vi "SetAdGain.vi"(1 "gain":u8) -> ()   [LabVIEW 2014]
uses:
  ESLSCDLL.dll
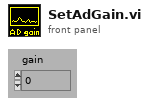
[diagram p1: front panel]
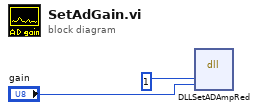
[diagram p0: block diagram]
diagram:
  n1 = dll-call lib="C:/Users/Gerhard/Documents/New64/lv/1cam/board.vis/ESLSCDLL.dll" fn="DLLSetADAmpRed"("drv"=u32 1, "gain"="gain") -> ()  [unwired: 6 in, 2 out]
